vi "Apply.vi"(8 "error in":errorcluster, 11 "HSU MCU V2 in":refnum<class "HSU MCU V2 CFG.lvclass">) -> (0 "error out":errorcluster, 3 "HSU MCU V2 out":refnum<class "HSU MCU V2 CFG.lvclass">)   [LabVIEW 2023, in "HSU MCU V2 CFG.lvclass"]
uses:
  HSU MCU V2 CFG.lvclass
  HSU MCU V2 CFG.lvclass/HSU MCU V2 CFG.ctl
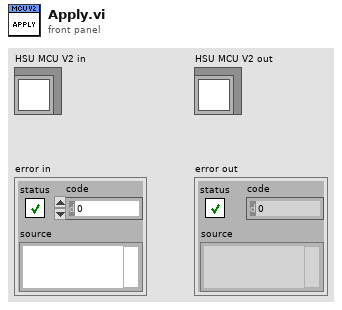
[diagram p1: front panel]
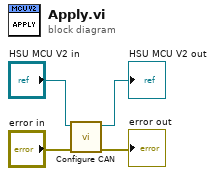
[diagram p0: block diagram]
diagram:
  n1 = call "Configure CAN.vi"("error in"="error in", "HSU MCU V2 Monitor CFG in"="HSU MCU V2 in") -> ("error out"=→"error out":errorcluster, "HSU MCU V2 Monitor CFG out"=→"HSU MCU V2 out":refnum<class "HSU MCU V2 CFG.lvclass">)  [unwired: 8 in]
